vi "Write Sweep Rate.vi"(8 "error in (no error)":errorcluster, 9 "Ramping Mode":T1, 10 "rate":dbl[unit] caption="Rate", 11 "Power Supply in":refnum<class "Power Supply.lvclass">) -> (0 "error out":errorcluster, 3 "Power Supply out":refnum<class "Power Supply.lvclass">)   [LabVIEW 2009, in "Power Supply.lvclass"]
uses:
  Power Supply.lvclass
  Ramping Mode.ctl
  Power Supply.lvclass/Power Supply.ctl
panel:
  out "rateok":bool
  out "maxrate":dbl[unit]
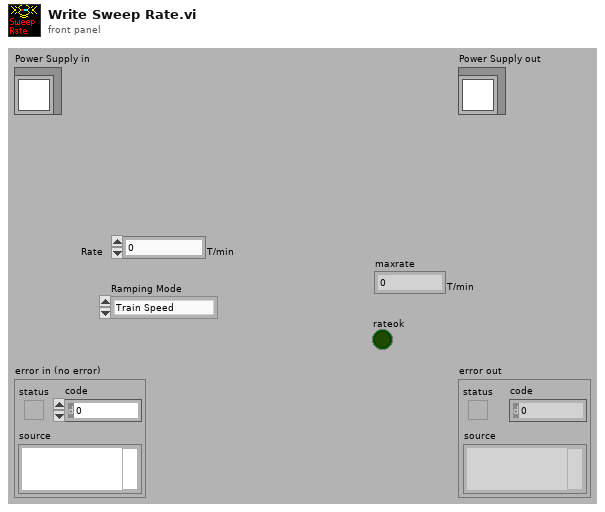
[diagram p1: front panel]
types:
  T1 = typedef "Power Supply.lvclass/Ramping Mode.ctl" = enum16{"Train Speed", "Maximum Speed", "Manual"}
  T2 = typedef "PSIO.ctl" = cluster{"Address":T3, "Version":enum16{"PS", "IPS"}}
  T3 = typedef "OxfordAddress.ctl" = cluster{"Com Port":i32, "ISOBUS Address":i32, "GPIB Address":i16, "Communication":enum16{"RS232", "ISOBUS", "GPIB", "Gateway"}}
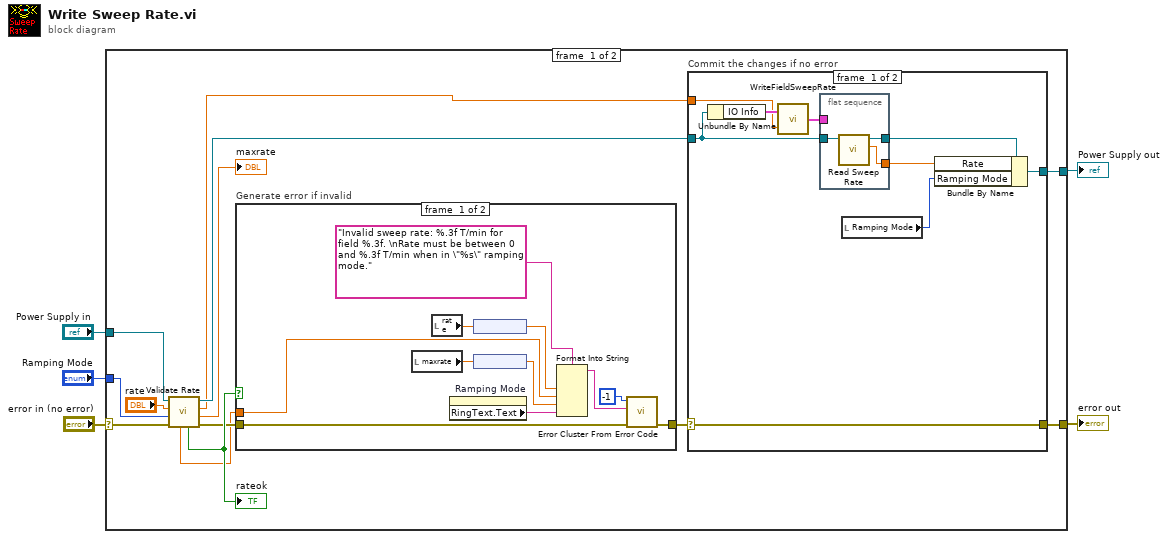
[diagram p0: block diagram]
diagram:
  n1 = case shown="No Error" "error in (no error)" {
    selector: "error in (no error)" -> [w12 w45]
    tunnel: [w18 w46] -> w5
    tunnel: [w15 w45] -> w1
    tunnel: "Power Supply in" -> [w14 w46]
    tunnel: "Ramping Mode" -> [w9 _]
    frame #0 {
      n2 = call "Validate Rate.vi"("error IO"=w12, "Ramping Mode"=w9, "rate"="rate", "Power Supply in"=w14) -> ("error out"=w11:errorcluster, "Max rate"=→"maxrate":dbl[unit], "Coerced rate"=w6:dbl[unit], "Power Supply out"=w13:refnum<class "Power Supply.lvclass">, "Coerced?"=w16:bool, "Field"=w10:dbl[unit])  [unwired: 2 in]
      "rateok" <- w16
      n3 = case "Generate error if invalid" shown="False" w16 {
        tunnel: [w43 w44] -> w17
        tunnel: w11 -> [w39 w44]
        tunnel: w10 -> [w37 _]
        frame #0 {
          n4 = local read "maxrate"() -> (w38:dbl[unit])
          n5 = local read "rate"() -> (w35:dbl[unit])
          n6 = property on="Ramping Mode" class="Enum (strict)"() -> ("RingText.Text"=w36:string)  [unwired: 2 in, 2 out]
          n7 = node(w35) -> (w34:dbl)
          n8 = node(w38) -> (w33:dbl)
          n9 = Format Into String(format string="Invalid sweep rate: %.3f T/min for field %.3f. \nRate must be between 0 and %.3f T/min when in \"%s\" ramping mode.", w34, w37, w33, w36) -> (resulting string=w41:string)  [unwired: 2 in, 1 out]
          n10 = call <vilib>:"Error Cluster From Error Code.vi"("error in (no error)"=w39, "error message (\"\")"=w41, "error code (0)"=-1) -> ("error out"=w43:errorcluster)  [unwired: 6 in]
        }
        frame #1 {
        }
      }
      n11 = case "Commit the changes if no error" shown="No Error" w17 {
        selector: w17 -> [w27 w32]
        tunnel: w6 -> [w24 _]
        tunnel: [w27 w32] -> w15
        tunnel: w13 -> [w21 w31]
        tunnel: [w25 w31] -> w18
        frame #0 {
          n12 = Unbundle By Name(w21) -> ("IO Info"=w26:T2)
          n13 = call "WriteFieldSweepRate.vi"("Sweep rate"=w24, "IO Info"=w26) -> ("IO Info"=w19:T2)
          n14 = flat-sequence {
            tunnel: [w30] -> w23
            tunnel: w21 -> [w29]
            tunnel: [w28] -> w20
            tunnel: w19 -> [_]
            frame #0 {
              n15 = call-dynamic "Read Sweep Rate.vi"("Power Supply in"=w29) -> ("Field sweep rate"=w30:dbl[unit], "Power Supply out"=w28:refnum<class "Power Supply.lvclass">)  [unwired: 8 in, 1 out]
            }
          }
          n16 = local read "Ramping Mode"() -> (w22:T1)
          n17 = Bundle By Name(cluster=w20, "Rate"=w23, "Ramping Mode"=w22) -> (w25:refnum<class "Power Supply.lvclass">)
        }
        frame #1 {
        }
      }
    }
    frame #1 {
    }
  }
  "Power Supply out" <- w5
  "error out" <- w1
